vi "PH_SSAC.BG File.vi"(0 "i ref in":refnum<vi>, 5 "error in":errorcluster) -> (14 "i ref out":refnum<vi>, 17 "BG File":path, 19 "error out":errorcluster)   [LabVIEW 2014, in "PH_SSAC.lvlib"]
doc: "This VI gets the name of the BG File."
uses:
  PH_SSAC.lvlib
  CSCore/CSSystem/CSSystemLib/CSSystemLib.lvlib
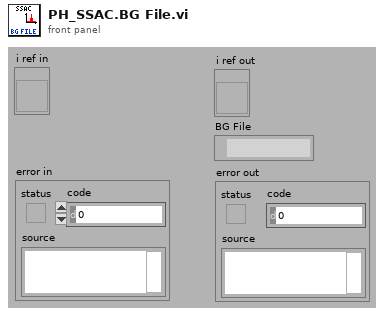
[diagram p1: front panel]
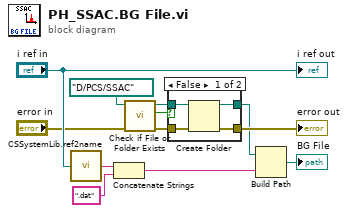
[diagram p0: block diagram]
diagram:
  n1 = call "CSSystemLib.ref2name.vi"("obj refnum"="i ref in") -> ("name"=w9:string)
  n2 = Concatenate Strings(w9, ".dat" ("string")) -> (w7:string)
  n3 = call <vilib>:"Check if File or Folder Exists.vi"("error in (no error)"="error in", "path"=path "D:/PCS/SSAC" ("base path")) -> ("error out"=w4:errorcluster, "file or folder exists?"=w6:bool, "dup path"=w3:path)  [unwired: 7 in]
  n4 = case shown="False" w6 {
    tunnel: w4 -> [w15 w17]
    tunnel: w3 -> [w16 w18]
    tunnel: [w13 w18] -> w2
    tunnel: [w14 w17] -> w12
    frame False {
      n5 = Create Folder(path (use dialog)=w16, error in=w15) -> (created path=w13:path, error out=w14:errorcluster)  [unwired: 1 in, 1 out]
    }
    frame True {
    }
  }
  "error out" <- w12
  n6 = Build Path(base path=w2, name or relative path=w7) -> (appended path=→"BG File":path)
  "i ref out" <- "i ref in"
